vi "Day04-2.vi"() -> ()   [LabVIEW 2021]
uses:
  <vilib>/Utility/error.llb/whitespace.ctl
panel:
  out "Array":i32[][](array[numeric])
  out "Answer":i32
  out "Bingo Numbers":string[](array[string])
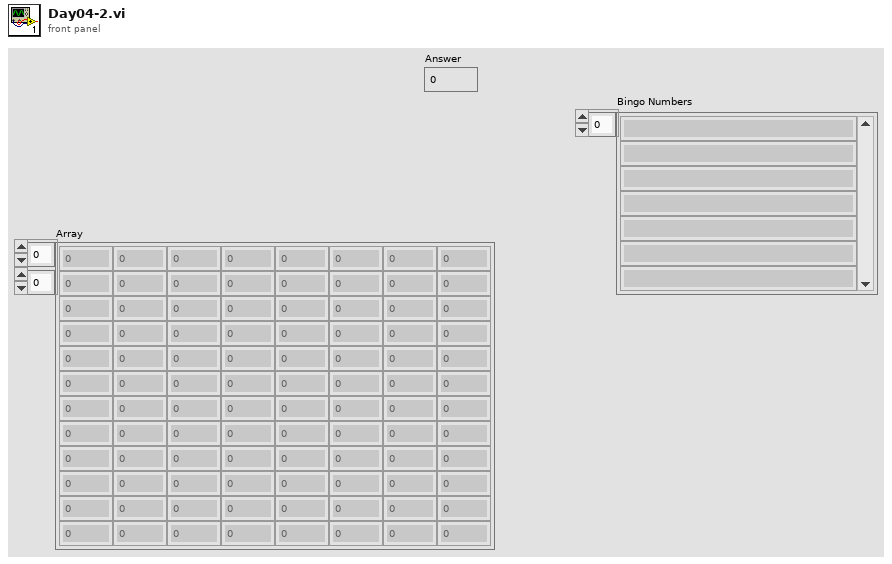
[diagram p1: front panel]
types:
  T1 = typedef "whitespace.ctl" = u16
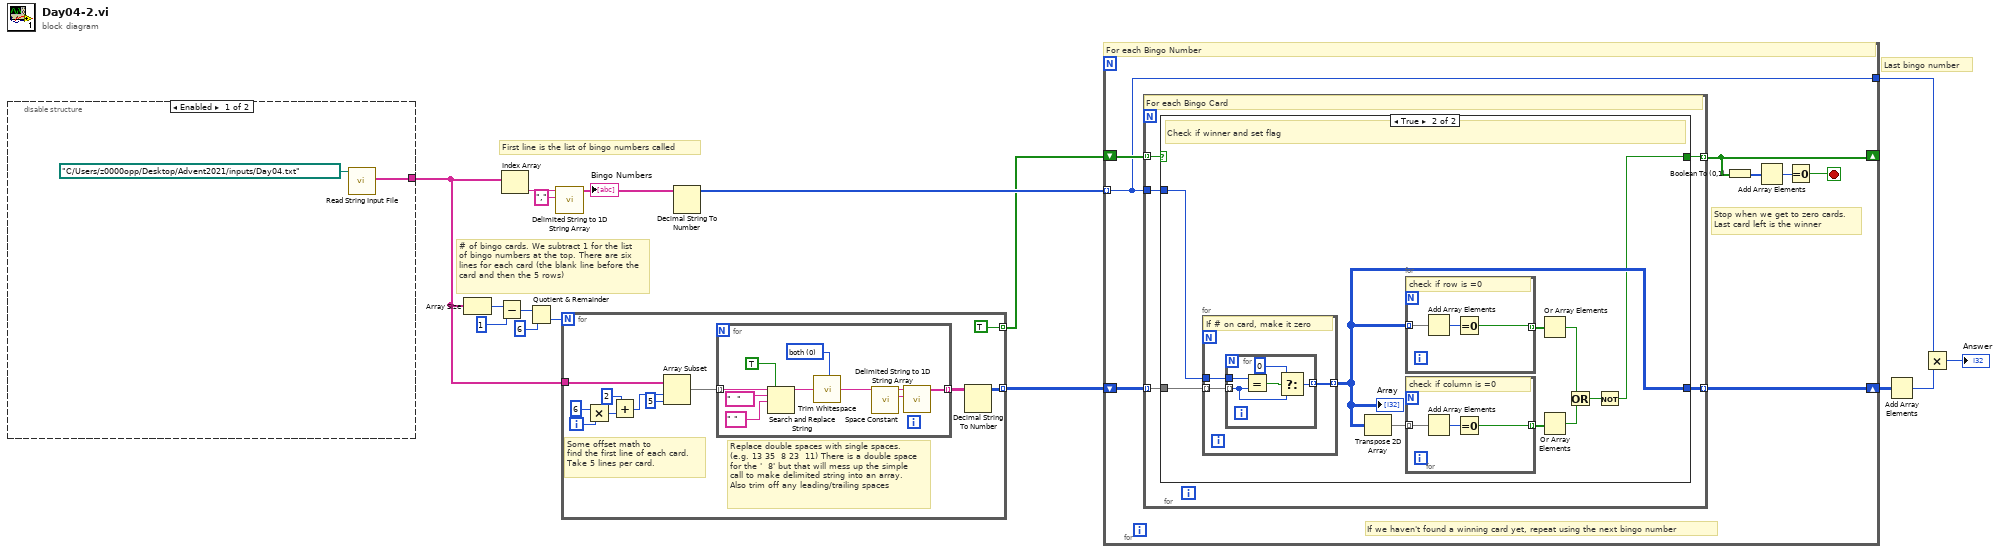
[diagram p0: block diagram]
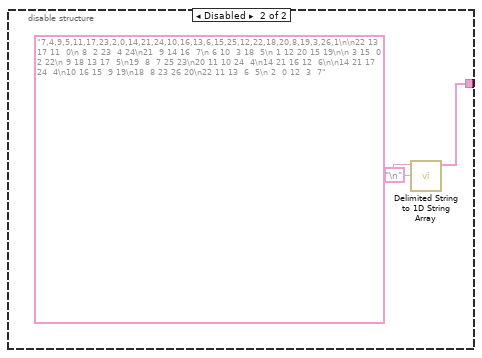
[diagram p2: hidden frame]
diagram:
  # "Last bingo number"
  # "# of bingo cards. We subtract 1 for the list of bingo numbers at the top. There are six lines for each card (the blank line before the card and then the 5 rows)"
  # "First line is the list of bingo numbers called"
  n1 = disable-structure shown="Enabled" {
    disable-tunnel: [w17 w19] -> w14
    frame Enabled {
      n2 = call "Read String Input File.vi"("file path (dialog if empty)"=path "C:/Users/z0000opp/Desktop/Advent2021/inputs/Day04.txt") -> ("input values"=w17:string[])  [unwired: 10 in]
    }
    frame Disabled {
      n3 = call <vilib>:"Delimited String to 1D String Array.vi"("delimiter"="\n", "delimited string"="7,4,9,5,11,17,23,2,0,14,21,24,10,16,13,6,15,25,12,22,18,20,8,19,3,26,1\n\n22 13 17 11  0\n 8  2 23  4 24\n21  9 14 16  7\n 6 10  3 18  5\n 1 12 20 15 19\n\n 3 15  0  2 22\n 9 18 13 17  5\n19  8  7 25 23\n20 11 10 24  4\n14 21 16 12  6\n\n14 21 17 24  4\n10 16 15  9 19\n18  8 23 26 20\n22 11 13  6  5\n 2  0 12  3  7") -> ("string array"=w19:string[])  [unwired: 9 in]
    }
  }
  n4 = Array Size(array=w14) -> (size(s)=w13:i32)
  n5 = Subtract(x=w13, y=1) -> (x-y=w11:i32)
  n6 = Index Array(array=w14) -> (element=w16:string)  [unwired: 1 in]
  n7 = Quotient & Remainder(x=w11, y=6) -> (floor(x/y)=w9:i32)  [unwired: 1 out]
  n8 = call <vilib>:"Delimited String to 1D String Array.vi"("delimiter"=",", "delimited string"=w16) -> ("string array"=w8:string[])  [unwired: 9 in]
  "Bingo Numbers" <- w8
  n9 = for {
    N: w9 -> [_]
    tunnel: w14 -> [w32]
    tunnel: [w23] -> w7 mode=indexing
    tunnel: [TRUE] -> w5 mode=indexing
    i -> [w31]
    # "Replace double spaces with single spaces.\n(e.g. 13 35  8 23  11) There is a double space\nfor the '  8' but that will mess up the simple\ncall to make delimited string into an array.\nAlso trim off any leading/trailing spaces"
    # "Some offset math to\nfind the first line of each card.\nTake 5 lines per card."
    n10 = Multiply(x=6, y=w31) -> (x*y=w29:i32)
    n11 = Add(x=2, y=w29) -> (x+y=w27:i32)
    n12 = Array Subset(array=w32, index=w27, length=5) -> (w26:string[])
    n13 = for {
      tunnel: w26 -> [w40] mode=indexing
      tunnel: [w41] -> w24 mode=indexing
      w33 = T1 0 items=["both", "start of string", "end of string"] ("location (both)")
      n14 = Search and Replace String(replace all?=TRUE ("replace all? (F)"), input string=w40, search string="  ", replace string=" ") -> (result string=w36:string)  [unwired: 4 in, 3 out]
      n15 = call <vilib>:"Trim Whitespace.vi"("string"=w36, "location (both)"=w33) -> ("trimmed string"=w34:string)
      n16 = call <vilib>:"Space Constant.vi"() -> ("String"=w35:string)
      n17 = call <vilib>:"Delimited String to 1D String Array.vi"("delimiter"=w35, "delimited string"=w34) -> ("string array"=w41:string[])  [unwired: 9 in]
    }
    n18 = Decimal String To Number(string=w24) -> (number=w23:i32[][])  [unwired: 2 in, 1 out]
  }
  n19 = Decimal String To Number(string=w8) -> (number=w6:i32[])  [unwired: 2 in, 1 out]
  n20 = for {
    tunnel: w6 -> [w43] mode=indexing
    shift-right: [w48] -> w4
    shift-left: w7 -> [w49]
    shift-right: [w46] -> _
    shift-left: w5 -> [w47]
    tunnel: [w43] -> w2
    stop <- w44 stop-if-true
    # "Stop when we get to zero cards.\nLast card left is the winner"
    # "If we haven't found a winning card yet, repeat using the next bingo number"
    # "For each Bingo Number"
    n21 = for {
      tunnel: w49 -> [w54] mode=indexing
      tunnel: w43 -> [w53]
      tunnel: [w52] -> w48 mode=indexing
      tunnel: w47 -> [w51] mode=indexing
      tunnel: [w50] -> w46 mode=indexing
      # "For each Bingo Card"
      n22 = case shown="True" w51 {
        selector: w51 -> [w55 _]
        tunnel: w54 -> [_ w65]
        tunnel: w53 -> [_ w59]
        tunnel: [_ w58] -> w52
        tunnel: [w55 w56] -> w50
        frame False {
          # "Already a winner, don't need to do anything"
        }
        frame True {
          # "Check if winner and set flag"
          n23 = for {
            tunnel: w65 -> [w74] mode=indexing
            tunnel: w59 -> [w73]
            tunnel: [w72] -> w58 mode=indexing
            # "If # on card, make it zero"
            n24 = for {
              tunnel: w74 -> [w77] mode=indexing
              tunnel: w73 -> [w79]
              tunnel: [w76] -> w72 mode=indexing
              n25 = Equal?(x=w79, y=w77) -> (x = y?=w78:bool)
              n26 = Select(t=0, s=w78, f=w77) -> (s? t:f=w76:i32)
            }
          }
          "Array" <- w58
          n27 = Transpose 2D Array(2D array=w58) -> (transposed array=w64:i32[][])
          n28 = for {
            tunnel: w58 -> [w71] mode=indexing
            tunnel: [w69] -> w63 mode=indexing
            # "check if row is =0"
            n29 = Add Array Elements(numeric array=w71) -> (sum=w70:i32)
            n30 = Equal To 0?(x=w70) -> (x = 0?=w69:bool)
          }
          n31 = for {
            tunnel: w64 -> [w68] mode=indexing
            tunnel: [w66] -> w62 mode=indexing
            # "check if column is =0"
            n32 = Add Array Elements(numeric array=w68) -> (sum=w67:i32)
            n33 = Equal To 0?(x=w67) -> (x = 0?=w66:bool)
          }
          n34 = Or Array Elements(Boolean array=w63) -> (logical OR=w60:bool)
          n35 = Or Array Elements(Boolean array=w62) -> (logical OR=w61:bool)
          n36 = Or(x=w60, y=w61) -> (x .or. y?=w57:bool)
          n37 = Not(x=w57) -> (.not. x?=w56:bool)
        }
      }
    }
    n38 = Boolean To (0,1)(Boolean=w46) -> (0, 1=w45:i16[])
    n39 = Add Array Elements(numeric array=w45) -> (sum=w42:i16)
    n40 = Equal To 0?(x=w42) -> (x = 0?=w44:bool)
  }
  n41 = Add Array Elements(numeric array=w4) -> (sum=w3:i32)
  n42 = Multiply(x=w2, y=w3) -> (x*y=→"Answer":i32)
